vi "Digital I_O.vi"() -> ()   [LabVIEW 2025]
panel:
  in  "Pin_DIN":u8=4 min=4 max=40
  out "error out":errorcluster
  out "Valor":bool
  in  "Pin_DOUT":u8=4 min=4 max=40
  in  "stop":bool
  in  "VISA resource name":refnum<visa-resource-name>
  # "Ejemplo: Lectura y escritura digital\nEste ejemplo muestra cómo utilizar las funciones de entrada y salida digital en LV_ESP32, permitiendo leer el estado de un pin digital y controlar la señal de salida en otro pin.\n\nEntradas requeridas:\nPin_DIN: Pin del que se leerá el estado digital (0 o 1).\nPin_DOUT: Pin en el que se enviará la señal digital.\n\nSalidas generadas:\nValor: Estado lógico que se desea aplicar al pin de salida (0 o 1).\nEstado leído del pin digital de entrada."
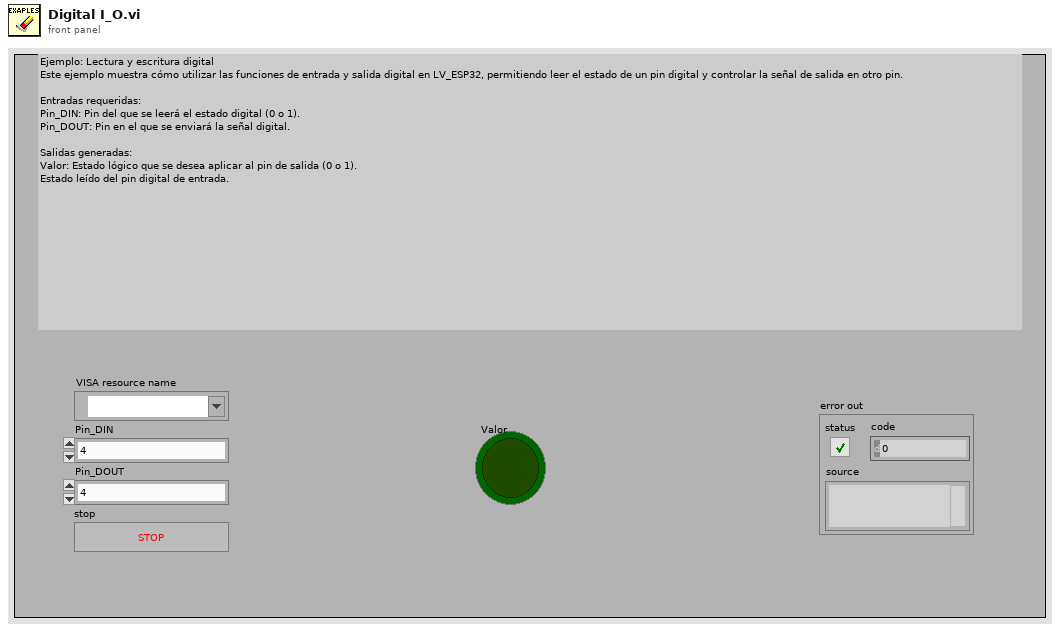
[diagram p1: front panel]
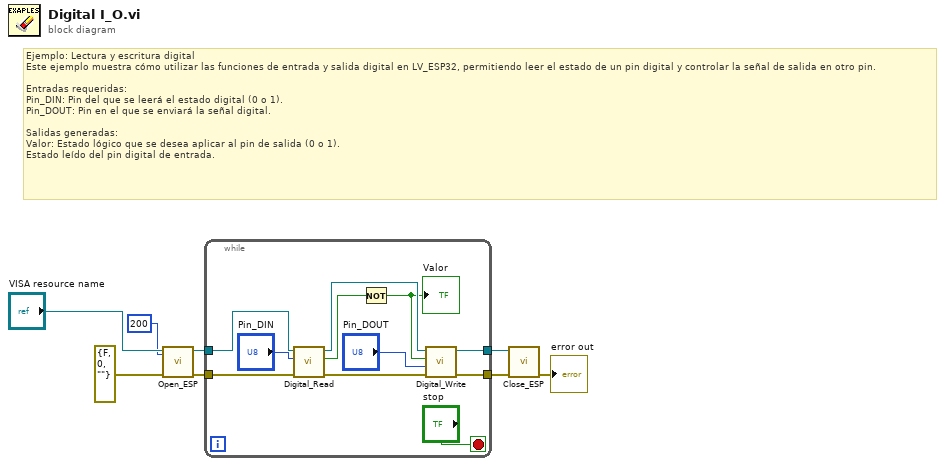
[diagram p0: block diagram]
diagram:
  # "Ejemplo: Lectura y escritura digital\nEste ejemplo muestra cómo utilizar las funciones de entrada y salida digital en LV_ESP32, permitiendo leer el estado de un pin digital y controlar la señal de salida en otro pin.\n\nEntradas requeridas:\nPin_DIN: Pin del que se leerá el estado digital (0 o 1).\nPin_DOUT: Pin en el que se enviará la señal digital.\n\nSalidas generadas:\nValor: Estado lógico que se desea aplicar al pin de salida (0 o 1).\nEstado leído del pin digital de entrada."
  n1 = call "Open_ESP.vi"("timeout (10sec)"=u32 200, "error in (no error)"=errorcluster {"status"=FALSE, "code"=0, "source"=""}, "VISA resource name"="VISA resource name") -> ("error out"=w6:errorcluster, "VISA resource name out"=w7:refnum<visa-resource-name>)  [unwired: 7 in]
  n2 = while {
    tunnel: w7 -> [w19]
    tunnel: w6 -> [w12]
    tunnel: [w17] -> w4
    tunnel: [w16] -> w3
    stop <- "stop" stop-if-true
    n3 = call "Digital_Read.vi"("error in (no error)"=w12, "Pin"="Pin_DIN", "VISA resource name"=w19) -> ("error out"=w15:errorcluster, "Valor"=w10:bool, "VISA resource name out"=w14:refnum<visa-resource-name>)  [unwired: 6 in]
    n4 = Not(x=w10) -> (.not. x?=w9:bool)
    "Valor" <- w9
    n5 = call "Digital_Write.vi"("error in (no error)"=w15, "Pin"="Pin_DOUT", "Estado"=w9, "VISA resource name"=w14) -> ("error out"=w16:errorcluster, "VISA resource name out"=w17:refnum<visa-resource-name>)  [unwired: 6 in]
  }
  n6 = call "Close_ESP.vi"("error in (no error)"=w3, "VISA resource name"=w4) -> ("error out"=→"error out":errorcluster)  [unwired: 9 in]
